vi "Digital IO polymorphe.vi"() -> ()   [LabVIEW 2020]
uses:
  <userlib>/DAQNavi Polymorphic VI/create/DAQNavi Create Channel(DO-Digital Output).vi
  <userlib>/DAQNavi Polymorphic VI/create/DAQNavi Create Channel(DI-Digital Input).vi
  <userlib>/DAQNavi Polymorphic VI/write/DAQNavi Write (Digital U8 1Chan 1Samp).vi
  <userlib>/DAQNavi Polymorphic VI/read/DAQNavi Read (Digital U8 1Chan 1Samp).vi
panel:
  in  "Stop":bool
  out "DI Read":u8
  out "DO Read":u8
  in  "DO Command":u8
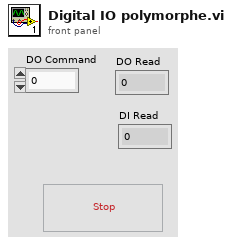
[diagram p1: front panel]
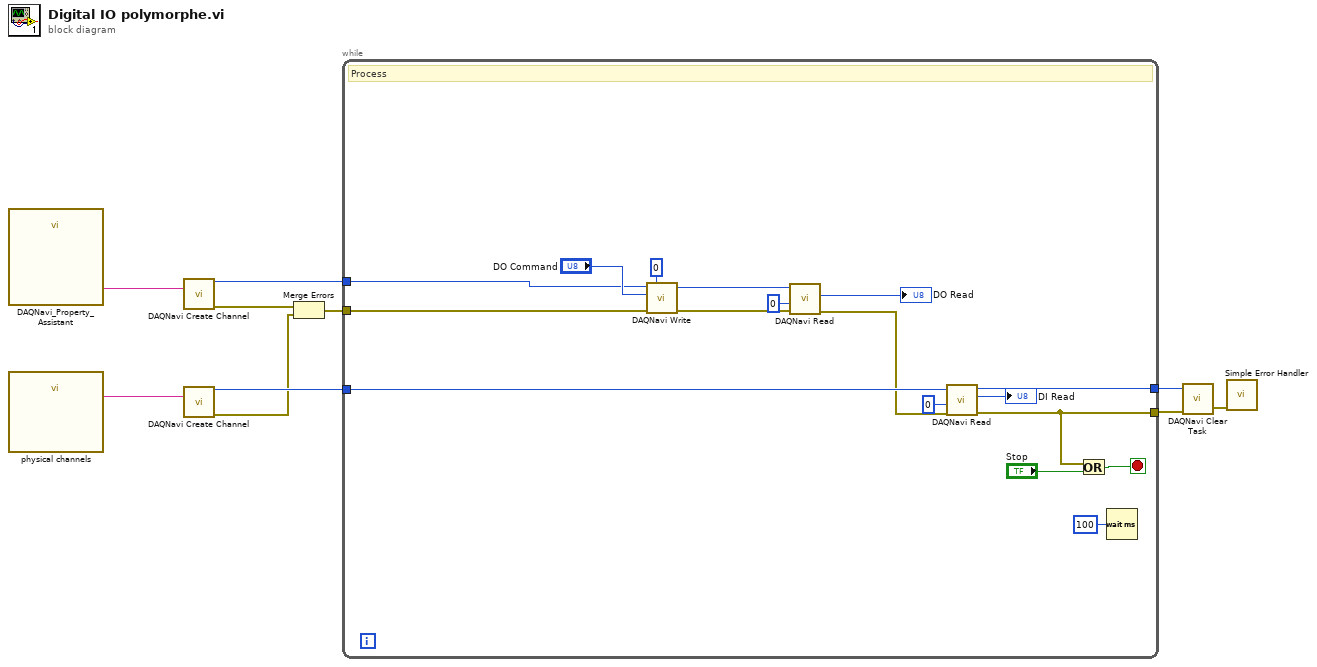
[diagram p0: block diagram]
diagram:
  n1 = call "DAQNavi_Property_Assistant"() -> ("property value"=w10:string)  [unwired: 1 in]
  n2 = call "physical channels"() -> ("property value"=w5:string)  [unwired: 1 out]
  n3 = call-poly <userlib>:"DAQNavi Create Channel.vi"("physical channels"=w10) -> ("task out"=w1:i32, "error out"=w4:errorcluster)  [unwired: 13 in]
  n4 = call-poly <userlib>:"DAQNavi Create Channel.vi"("physical channels"=w5) -> ("task out"=w6:i32, "error out"=w2:errorcluster)  [unwired: 4 in, 9 out]
  n5 = Merge Errors(w4, w2) -> (w3:errorcluster)
  n6 = while {
    tunnel: w6 -> [w27]
    tunnel: [w26] -> w8
    tunnel: [w20] -> w7
    tunnel: w3 -> [w12]
    tunnel: w1 -> [w11]
    stop <- w24 stop-if-true
    # "Process"
    n7 = call-poly <userlib>:"DAQNavi Write.vi"("portBit"=0, "error in (no error)"=w12, "data"="DO Command", "task in"=w11) -> ("error out"=w18:errorcluster, "task out"=w19:i32)  [unwired: 5 in, 1 out]
    n8 = call-poly <userlib>:"DAQNavi Read.vi"("error in (no error)"=w18, "portBit"=0, "task in"=w19) -> ("error out"=w13:errorcluster, "data"=→"DO Read":u8)  [unwired: 1 in, 6 out]
    n9 = call-poly <userlib>:"DAQNavi Read.vi"("error in (no error)"=w13, "portBit"=0, "task in"=w27) -> ("error out"=w20:errorcluster, "data"=→"DI Read":u8, "task out"=w26:i32)  [unwired: 1 in, 5 out]
    n10 = Or(x=w20, y="Stop") -> (x .or. y?=w24:bool)
    n11 = Wait (ms)(milliseconds to wait=u32 100) -> ()  [unwired: 1 out]
  }
  n12 = call <userlib>:"DAQNavi Clear Task.vi"("error in (no error)"=w7, "task in"=w8) -> ("error out"=w9:errorcluster)  [unwired: 1 out]
  n13 = call <vilib>:"Simple Error Handler.vi"("error in (no error)"=w9) -> ()  [unwired: 2 in, 7 out]
